vi "array.vi"() -> ()   [LabVIEW 2018]
uses:
  <vilib>/Analysis/Matrix/Datatypes/RealMatrix.ctl
  <vilib>/Analysis/Matrix/NI_Matrix.lvlib
panel:
  in  "Array":bool[][](array[boolean])
  out "error in (no error) 2":errorcluster
  in  "Real Matrix":T1
  out "size(s)":i32[](array[numeric])
  out "appended array":dbl[][](array[numeric])
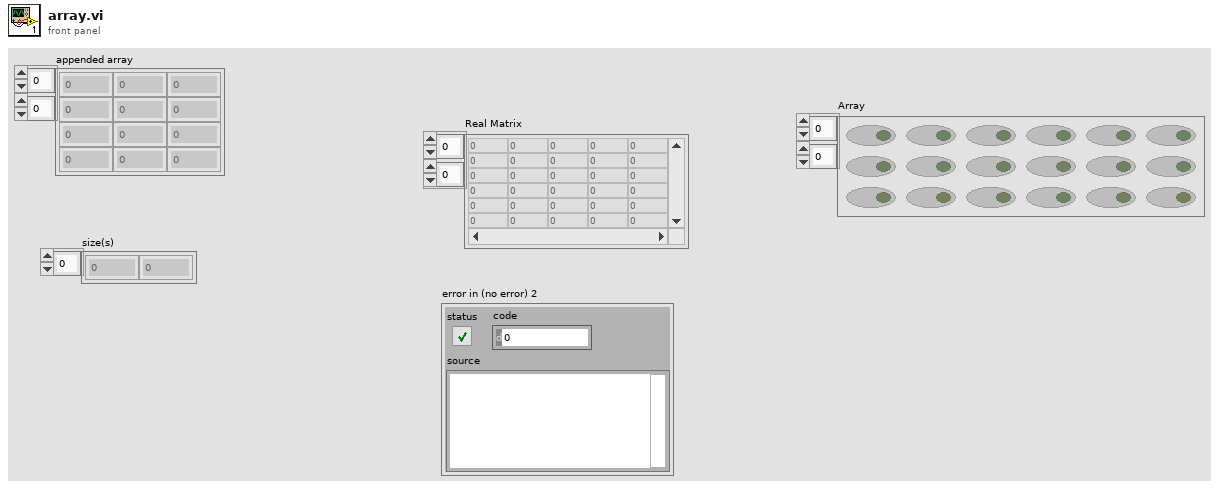
[diagram p1: front panel]
types:
  T1 = typedef "NI_Matrix.lvlib/RealMatrix.ctl" = dbl[][]
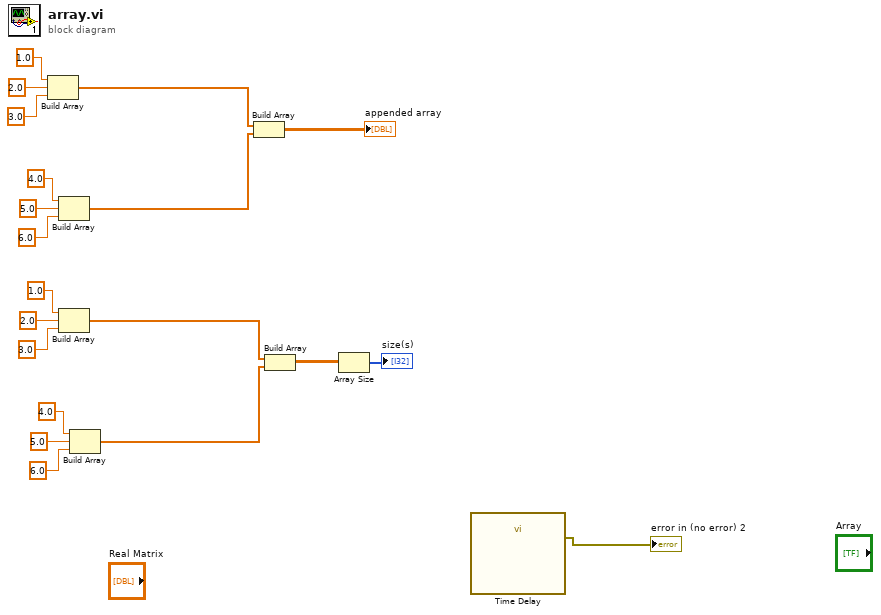
[diagram p0: block diagram]
diagram:
  n1 = Build Array(1.0 ("element"), 2.0 ("element"), 3.0 ("element")) -> (w14:dbl[])
  n2 = Build Array(4.0 ("element"), 5.0 ("element"), 6.0 ("element")) -> (w13:dbl[])
  n3 = Build Array(1.0 ("element"), 2.0 ("element"), 3.0 ("element")) -> (w5:dbl[])
  n4 = Build Array(4.0 ("element"), 5.0 ("element"), 6.0 ("element")) -> (w4:dbl[])
  n5 = Build Array(w14, w13) -> (→"appended array":dbl[][])
  n6 = Build Array(w5, w4) -> (w3:dbl[][])
  n7 = Array Size(array=w3) -> (size(s)=→"size(s)":i32[])
  n8 = call "Time Delay"() -> ("error out"=→"error in (no error) 2":errorcluster)  [unwired: 11 in]
